vi "CRYCal Harmonics Diff.vi"(0 "HT Option":bool[](array[boolean]), 1 "x":dbl[](array[numeric]), 2 "z":dbl[](array[numeric]), 3 "Index":i32, 5 "Method":u16, 7 "Harmonic":dbl[](array[numeric]), 9 "Freq resp curves":dbl[][](array[numeric]), 11 "Total Noise":dbl[](array[numeric]), 12 "Fs":dbl format="%.2f", 13 "max value1":dbl, 14 "max value2":dbl) -> (4 "Harmonic Track Out":T1(array[cluster]))   [LabVIEW 2013]
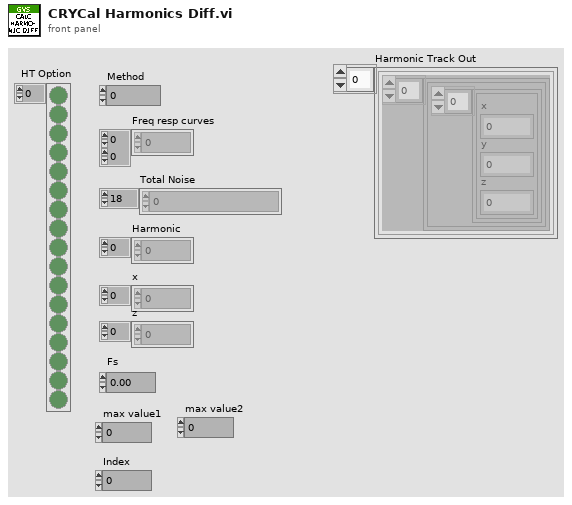
[diagram p1: front panel]
types:
  T1 = cluster{cluster{cluster{"x":dbl, "y":dbl, "z":dbl}[]}[]}[]
  T2 = cluster{cluster{"x":dbl, "Log Out":dbl, "Z":dbl}[]}
  T3 = cluster{cluster{"x":dbl, "Log Out":dbl, "Z":dbl}[]}[]
  T4 = cluster{"Freq resp curves clipped":cluster{cluster{"x":dbl, "y":dbl, "z":dbl}[]}[]}[]
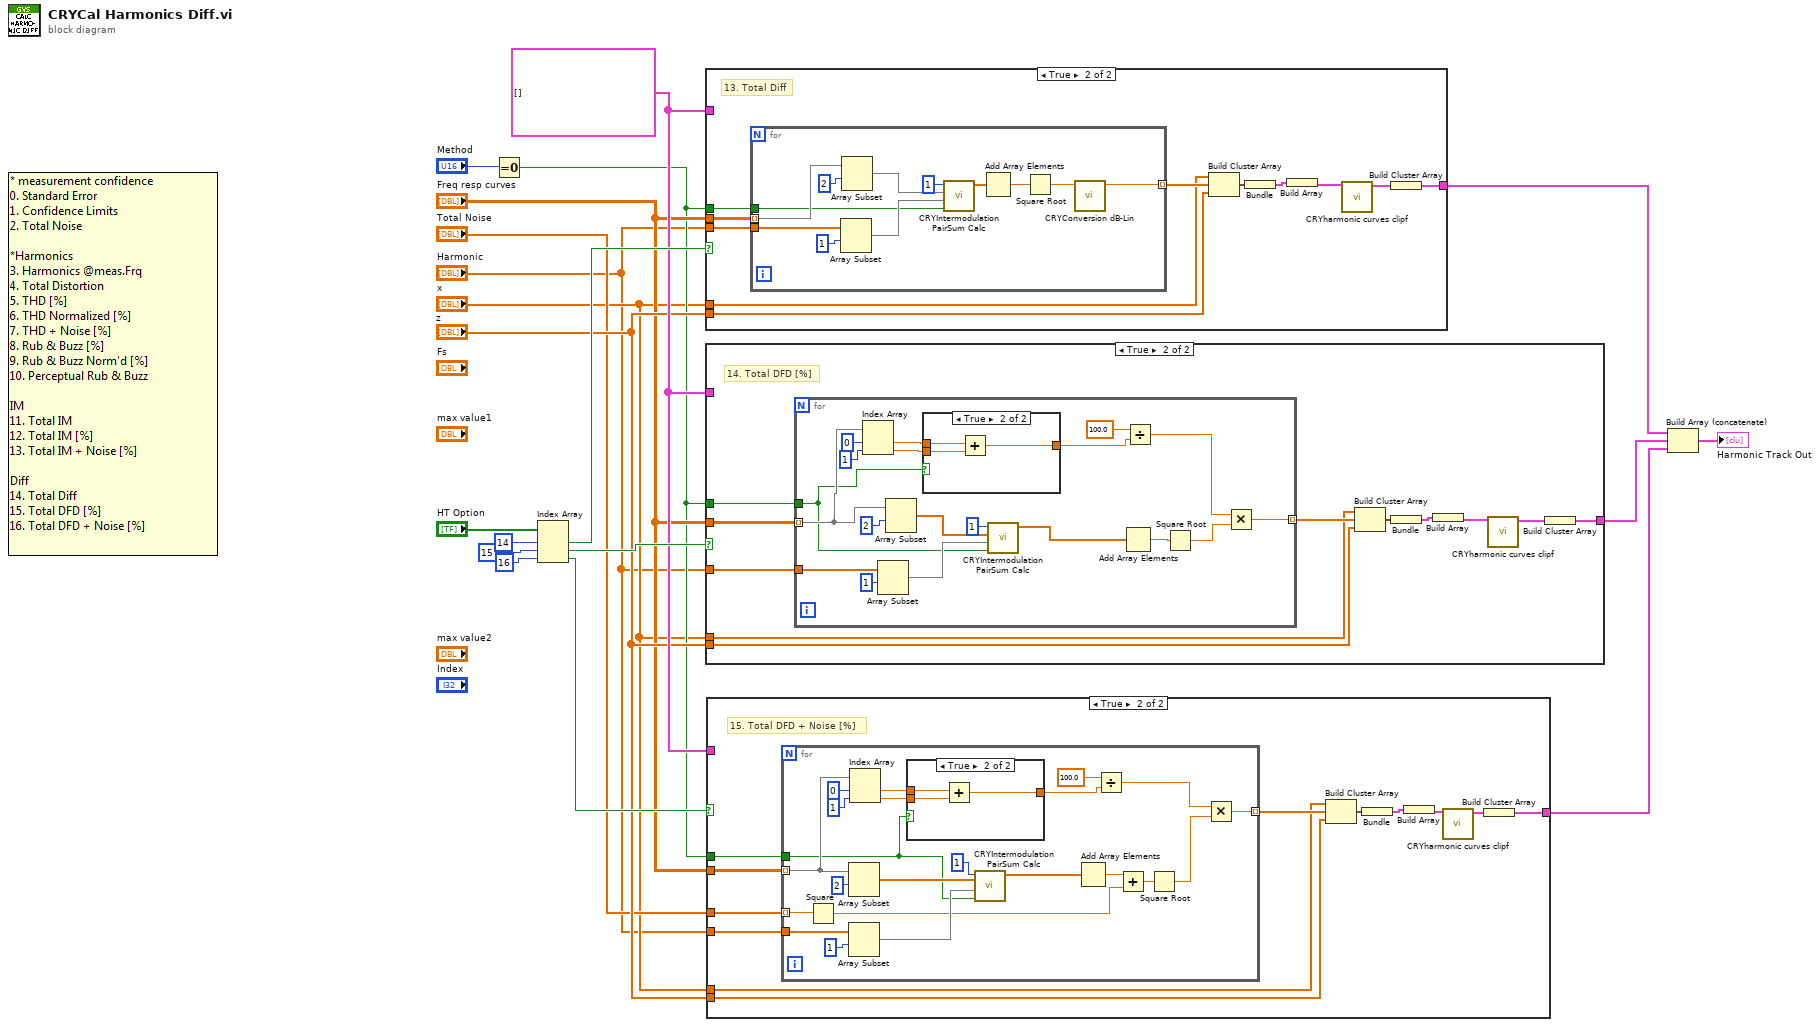
[diagram p0: block diagram]
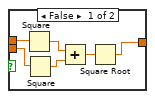
[diagram p3: hidden frame]
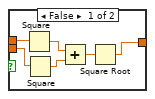
[diagram p5: hidden frame]
diagram:
  w7 = cluster{cluster{cluster[]}[]}[] []
  n1 = Equal To 0?(x="Method") -> (x = 0?=w3:bool)
  n2 = Index Array(array="HT Option", index #1=14 ("index"), index #2=15 ("index"), index #3=16 ("index")) -> (element #1=w13:bool, element #2=w12:bool, element #3=w11:bool)
  n3 = case shown="True" w13 {
    tunnel: [w20 w29] -> w10
    tunnel: "Freq resp curves" -> [_ w25]
    tunnel: "Harmonic" -> [_ w24]
    tunnel: w3 -> [_ w23]
    tunnel: "x" -> [_ w22]
    tunnel: "z" -> [_ w21]
    tunnel: w7 -> [w20 _]
    frame False {
    }
    frame True {
      # "13. Total Diff"
      n4 = for {
        tunnel: w25 -> [w40] mode=indexing
        tunnel: [w33] -> w28 mode=indexing
        tunnel: w24 -> [w43]
        tunnel: w23 -> [w32]
        n5 = Array Subset(array=w43, index=1) -> (w38:dbl[])  [unwired: 1 in]
        n6 = Array Subset(array=w40, index=2) -> (w37:dbl[])  [unwired: 1 in]
        n7 = call "CRYIntermodulation PairSum Calc.vi"("Is IEC?"=w32, "Order Array"=w38, "Data Array"=w37, "Type"=u32 1) -> ("PairSum Array"=w39:dbl[])  [unwired: 7 in]
        n8 = Add Array Elements(numeric array=w39) -> (sum=w35:dbl)
        n9 = Square Root(x=w35) -> (sqrt(x)=w34:dbl)
        n10 = call "CRYConversion dB-Lin.vi"("Lin In"=w34) -> ("Log Out"=w33:dbl)  [unwired: 5 in, 3 out]
      }
      n11 = Build Cluster Array(w22, w28, w21) -> (w30:cluster{"x":dbl, "Log Out":dbl, "Z":dbl}[])
      n12 = Bundle(w30) -> (w31:T2)  [unwired: 1 in]
      n13 = Build Array(w31) -> (w27:T3)
      n14 = call "CRYharmonic curves clipf.vi"("Freq resp curves"=w27) -> ("Freq resp curves clipped"=w26:cluster{cluster{"x":dbl, "y":dbl, "z":dbl}[]}[])  [unwired: 2 in, 8 out]
      n15 = Build Cluster Array(w26) -> (w29:T4)
    }
  }
  n16 = case shown="True" w12 {
    tunnel: [w44 w53] -> w9
    tunnel: w7 -> [w44 _]
    tunnel: "Freq resp curves" -> [_ w49]
    tunnel: w3 -> [_ w48]
    tunnel: "Harmonic" -> [_ w47]
    tunnel: "x" -> [_ w46]
    tunnel: "z" -> [_ w45]
    frame False {
    }
    frame True {
      # "14. Total DFD [%]"
      n17 = for {
        tunnel: w49 -> [w64] mode=indexing
        tunnel: [w62] -> w52 mode=indexing
        tunnel: w48 -> [w57]
        tunnel: w47 -> [w56]
        n18 = Index Array(array=w64, index #1=0 ("index"), index #2=1 ("index")) -> (element #1=w60:dbl, element #2=w59:dbl)
        n19 = Array Subset(array=w56, index=1) -> (w71:dbl[])  [unwired: 1 in]
        n20 = Array Subset(array=w64, index=2) -> (w70:dbl[])  [unwired: 1 in]
        n21 = case shown="True" w57 {
          tunnel: w60 -> [w80 w83]
          tunnel: w59 -> [w79 w82]
          tunnel: [w75 w81] -> w58
          frame False {
            n22 = Square(x=w80) -> (x^2=w78:dbl)
            n23 = Square(x=w79) -> (x^2=w77:dbl)
            n24 = Add(x=w78, y=w77) -> (x+y=w76:dbl)
            n25 = Square Root(x=w76) -> (sqrt(x)=w75:dbl)
          }
          frame True {
            n26 = Add(x=w83, y=w82) -> (x+y=w81:dbl)
          }
        }
        n27 = call "CRYIntermodulation PairSum Calc.vi"("Is IEC?"=w57, "Order Array"=w71, "Data Array"=w70, "Type"=u32 1) -> ("PairSum Array"=w72:dbl[])  [unwired: 7 in]
        n28 = Add Array Elements(numeric array=w72) -> (sum=w68:dbl)
        n29 = Divide(x=100.0, y=w58) -> (x/y=w61:dbl)
        n30 = Square Root(x=w68) -> (sqrt(x)=w63:dbl)
        n31 = Multiply(x=w61, y=w63) -> (x*y=w62:dbl)
      }
      n32 = Build Cluster Array(w46, w52, w45) -> (w54:cluster{"x":dbl, dbl, "Z":dbl}[])
      n33 = Bundle(w54) -> (w55:cluster{cluster{"x":dbl, dbl, "Z":dbl}[]})  [unwired: 1 in]
      n34 = Build Array(w55) -> (w51:cluster{cluster{"x":dbl, dbl, "Z":dbl}[]}[])
      n35 = call "CRYharmonic curves clipf.vi"("Freq resp curves"=w51) -> ("Freq resp curves clipped"=w50:cluster{cluster{"x":dbl, "y":dbl, "z":dbl}[]}[])  [unwired: 2 in, 8 out]
      n36 = Build Cluster Array(w50) -> (w53:T4)
    }
  }
  n37 = case shown="True" w11 {
    tunnel: [w84 w94] -> w8
    tunnel: w7 -> [w84 _]
    tunnel: "x" -> [_ w90]
    tunnel: "z" -> [_ w89]
    tunnel: "Freq resp curves" -> [_ w88]
    tunnel: "Harmonic" -> [_ w87]
    tunnel: "Total Noise" -> [_ w86]
    tunnel: w3 -> [_ w85]
    frame False {
    }
    frame True {
      # "15. Total DFD + Noise [%]"
      n38 = for {
        tunnel: w88 -> [w108] mode=indexing
        tunnel: [w106] -> w93 mode=indexing
        tunnel: w87 -> [w118]
        tunnel: w86 -> [w104] mode=indexing
        tunnel: w85 -> [w98]
        n39 = Square(x=w104) -> (x^2=w102:dbl)
        n40 = Array Subset(array=w108, index=2) -> (w113:dbl[])  [unwired: 1 in]
        n41 = Array Subset(array=w118, index=1) -> (w114:dbl[])  [unwired: 1 in]
        n42 = Index Array(array=w108, index #1=0 ("index"), index #2=1 ("index")) -> (element #1=w100:dbl, element #2=w99:dbl)
        n43 = case shown="True" w98 {
          tunnel: w100 -> [w124 w127]
          tunnel: w99 -> [w123 w126]
          tunnel: [w119 w125] -> w97
          frame False {
            n44 = Square(x=w124) -> (x^2=w122:dbl)
            n45 = Square(x=w123) -> (x^2=w121:dbl)
            n46 = Add(x=w122, y=w121) -> (x+y=w120:dbl)
            n47 = Square Root(x=w120) -> (sqrt(x)=w119:dbl)
          }
          frame True {
            n48 = Add(x=w127, y=w126) -> (x+y=w125:dbl)
          }
        }
        n49 = call "CRYIntermodulation PairSum Calc.vi"("Is IEC?"=w98, "Order Array"=w114, "Data Array"=w113, "Type"=u32 1) -> ("PairSum Array"=w115:dbl[])  [unwired: 7 in]
        n50 = Add Array Elements(numeric array=w115) -> (sum=w103:dbl)
        n51 = Divide(x=100.0, y=w97) -> (x/y=w105:dbl)
        n52 = Add(x=w103, y=w102) -> (x+y=w101:dbl)
        n53 = Square Root(x=w101) -> (sqrt(x)=w107:dbl)
        n54 = Multiply(x=w105, y=w107) -> (x*y=w106:dbl)
      }
      n55 = Build Cluster Array(w90, w93, w89) -> (w95:cluster{"x":dbl, dbl, "Z":dbl}[])
      n56 = Bundle(w95) -> (w96:cluster{cluster{"x":dbl, dbl, "Z":dbl}[]})  [unwired: 1 in]
      n57 = Build Array(w96) -> (w92:cluster{cluster{"x":dbl, dbl, "Z":dbl}[]}[])
      n58 = call "CRYharmonic curves clipf.vi"("Freq resp curves"=w92) -> ("Freq resp curves clipped"=w91:cluster{cluster{"x":dbl, "y":dbl, "z":dbl}[]}[])  [unwired: 2 in, 8 out]
      n59 = Build Cluster Array(w91) -> (w94:T4)
    }
  }
  n60 = Build Array (concatenate)(w10, w9, w8) -> (→"Harmonic Track Out":T4)
